vi "Unit Test Commands.vi"() -> ()   [LabVIEW 2015, in "PAS.lvclass"]
uses:
  PAS.lvclass
  Typedefs/Valves.ctl
  Typedefs/Emitter Power.ctl
panel:
  out "Write Success?":bool
  out "Finished Ramping?":bool
  out "Frequency":dbl
  out "ADC":dbl
  out "Temperature":dbl
  out "Serial Number":string
  out "Hardware Version":string
  out "Firmware Version":string
  out "Build Date":string
  out "Ready?":bool
  out "error out":errorcluster
  # "PAS Unit Test"
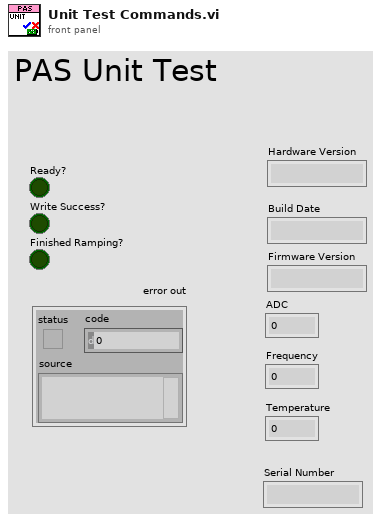
[diagram p1: front panel]
types:
  T1 = typedef "PAS.lvclass/Emitter Power.ctl" = u16
  T2 = typedef "PAS.lvclass/Valves.ctl" = u16
  T3 = typedef "PAS.lvclass/Session Handle.ctl" = refnum<data-value>
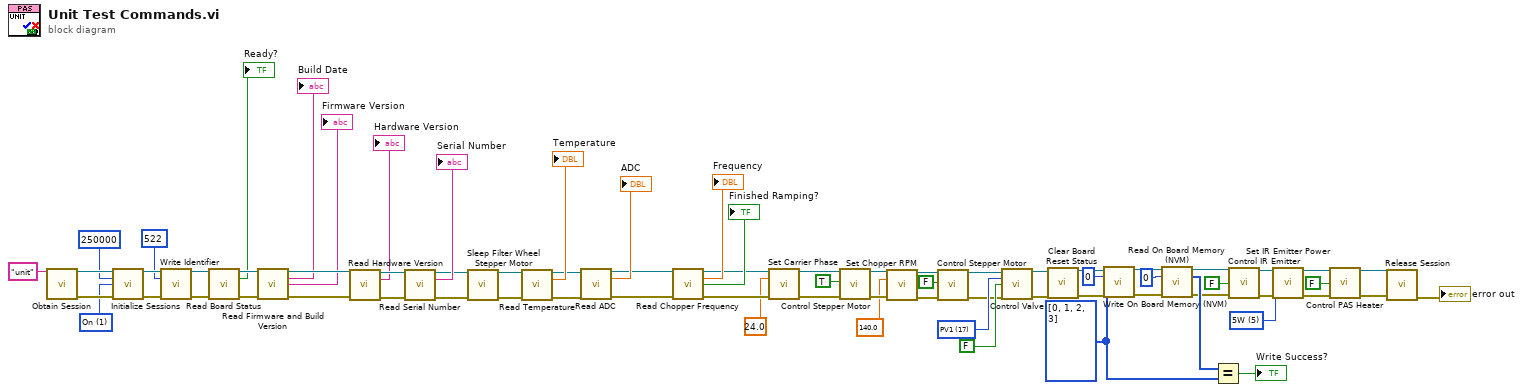
[diagram p0: block diagram]
diagram:
  w9 = u8[] [0, 1, 2, 3] ("Bytes to Write")
  w52 = T1 5 items=["2W"=2, "3W"=3, "4W"=4, "5W"=5] ("Emitter Power")
  w58 = T2 17 items=["PV1"=17, "PV2"=18, "PV3"=19, "PV4"=20] ("Valves")
  w68 = u32 1 items=["Off", "On"] ("Termination")
  n1 = call "Obtain Session.vi"("Session  Name ()"="unit") -> ("Session Handle"=w72:T3, "error out"=w71:errorcluster)  [unwired: 13 in]
  n2 = call "Initialize Sessions.vi"("Session Handle in"=w72, "Baud Rate"=u32 250000, "Termination"=w68, "error in (no error)"=w71) -> ("Session Handle Out"=w67:T3, "error out"=w66:errorcluster)  [unwired: 10 in]
  n3 = call "Write Identifier.vi"("Session Handle in"=w67, "identifier"=u16 522, "error in (no error)"=w66) -> ("Session Handle out"=w57:T3, "error out"=w56:errorcluster)  [unwired: 11 in]
  n4 = call "Read Board Status.vi"("Session Handle in"=w57, "error in (no error)"=w56) -> ("Session Handle out"=w55:T3, "Ready?"=→"Ready?":bool, "error out"=w54:errorcluster)  [unwired: 11 in]
  n5 = call "Read Firmware and Build Version.vi"("Session Handle in"=w55, "error in (no error)"=w54) -> ("Session Handle out"=w63:T3, "Build Date"=→"Build Date":string, "Firmware Version"=→"Firmware Version":string, "error out"=w62:errorcluster)  [unwired: 10 in]
  n6 = call "Read Hardware Version.vi"("Session Handle in"=w63, "error in (no error)"=w62) -> ("Session Handle out"=w61:T3, "Hardware Version"=→"Hardware Version":string, "error out"=w60:errorcluster)  [unwired: 11 in]
  n7 = call "Read Serial Number.vi"("Session Handle in"=w61, "error in (no error)"=w60) -> ("Session Handle out"=w42:T3, "Serial Number"=→"Serial Number":string, "error out"=w41:errorcluster)  [unwired: 11 in]
  n8 = call "Sleep Filter Wheel Stepper Motor.vi"("Session Handle in"=w42, "error in (no error)"=w41) -> ("Session Handle out"=w40:T3, "error out"=w39:errorcluster)  [unwired: 10 in, 2 out]
  n9 = call "Read Temperature.vi"("Session Handle in"=w40, "error in (no error)"=w39) -> ("Session Handle out"=w2:T3, "Temperature"=→"Temperature":dbl, "error out"=w1:errorcluster)  [unwired: 9 in, 2 out]
  n10 = call "Read ADC.vi"("Session Handle in"=w2, "error in (no error)"=w1) -> ("Session Handle out"=w35:T3, "ADC"=→"ADC":dbl, "error out"=w36:errorcluster)  [unwired: 9 in, 2 out]
  n11 = call "Read Chopper Frequency.vi"("Session Handle in"=w35, "error in (no error)"=w36) -> ("Session Handle out"=w32:T3, "Frequency"=→"Frequency":dbl, "Finished Ramping?"=→"Finished Ramping?":bool, "error out"=w31:errorcluster)  [unwired: 9 in, 1 out]
  n12 = call "Set Carrier Phase.vi"("Session Handle in"=w32, "Phase"=24.0, "error in (no error)"=w31) -> ("Session Handle out"=w29:T3, "error out"=w28:errorcluster)  [unwired: 10 in, 1 out]
  n13 = call "Control Stepper Motor.vi"("Session Handle in"=w29, "Start?"=TRUE, "error in (no error)"=w28) -> ("Session Handle out"=w26:T3, "error out"=w25:errorcluster)  [unwired: 10 in, 1 out]
  n14 = call "Set Chopper RPM.vi"("Session Handle in"=w26, "RPM"=140.0, "error in (no error)"=w25) -> ("Session Handle out"=w21:T3, "error out"=w22:errorcluster)  [unwired: 10 in, 1 out]
  n15 = call "Control Stepper Motor.vi"("Session Handle in"=w21, "Start?"=FALSE, "error in (no error)"=w22) -> ("Session Handle out"=w19:T3, "error out"=w20:errorcluster)  [unwired: 10 in, 1 out]
  n16 = call "Control Valve.vi"("Session Handle in"=w19, "Valves"=w58, "Energize?"=FALSE, "error in (no error)"=w20) -> ("Session Handle out"=w18:T3, "error out"=w17:errorcluster)  [unwired: 8 in, 2 out]
  n17 = call "Clear Board Reset Status.vi"("Session Handle in"=w18, "error in (no error)"=w17) -> ("Session Handle out"=w16:T3, "error out"=w15:errorcluster)  [unwired: 11 in, 1 out]
  n18 = call "Write On Board Memory (NVM).vi"("Session Handle in"=w16, "Address"=u16 0, "Bytes to Write"=w9, "error in (no error)"=w15) -> ("Session Handle out"=w13:T3, "error out"=w12:errorcluster)  [unwired: 10 in]
  n19 = call "Read On Board Memory (NVM).vi"("Session Handle in"=w13, "Address"=u16 0, "error in (no error)"=w12) -> ("Session Handle out"=w7:T3, "Read Bytes"=w10:u8[], "error out"=w5:errorcluster)  [unwired: 10 in]
  n20 = Equal?(x=w10, y=w9) -> (x = y?=→"Write Success?":bool)
  n21 = call "Control IR Emitter.vi"("Session Handle in"=w7, "Start?"=FALSE, "error in (no error)"=w5) -> ("Session Handle out"=w6:T3, "error out"=w4:errorcluster)  [unwired: 9 in, 2 out]
  n22 = call "Set IR Emitter Power.vi"("Session Handle in"=w6, "Emitter Power"=w52, "error in (no error)"=w4) -> ("Session Handle out"=w51:T3, "error out"=w50:errorcluster)  [unwired: 10 in, 1 out]
  n23 = call "Control PAS Heater.vi"("Session Handle in"=w51, "Start?"=FALSE, "error in (no error)"=w50) -> ("Session Handle out"=w48:T3, "error out"=w47:errorcluster)  [unwired: 9 in, 2 out]
  n24 = call "Release Session.vi"("Session Handle"=w48, "error in (no error)"=w47) -> ("error out"=→"error out":errorcluster)  [unwired: 13 in]
